vi "LV_webcam_image_analysis.vi"() -> ()   [LabVIEW 2014]
uses:
  <vilib>/userdefined/High Color/IMAQdx.ctl
  <vilib>/vision/driver/NI_Vision_Acquisition_Software.lvlib
  <vilib>/vision/NI_Vision_Development_Module.lvlib
panel:
  out "Boolean 2":bool
  out "Boolean":bool
  out "Color Spectrum":dbl[](array[numeric]) format="%.2f"
  out "Image":T1(plugin-control)
  in  "Stop Button":bool
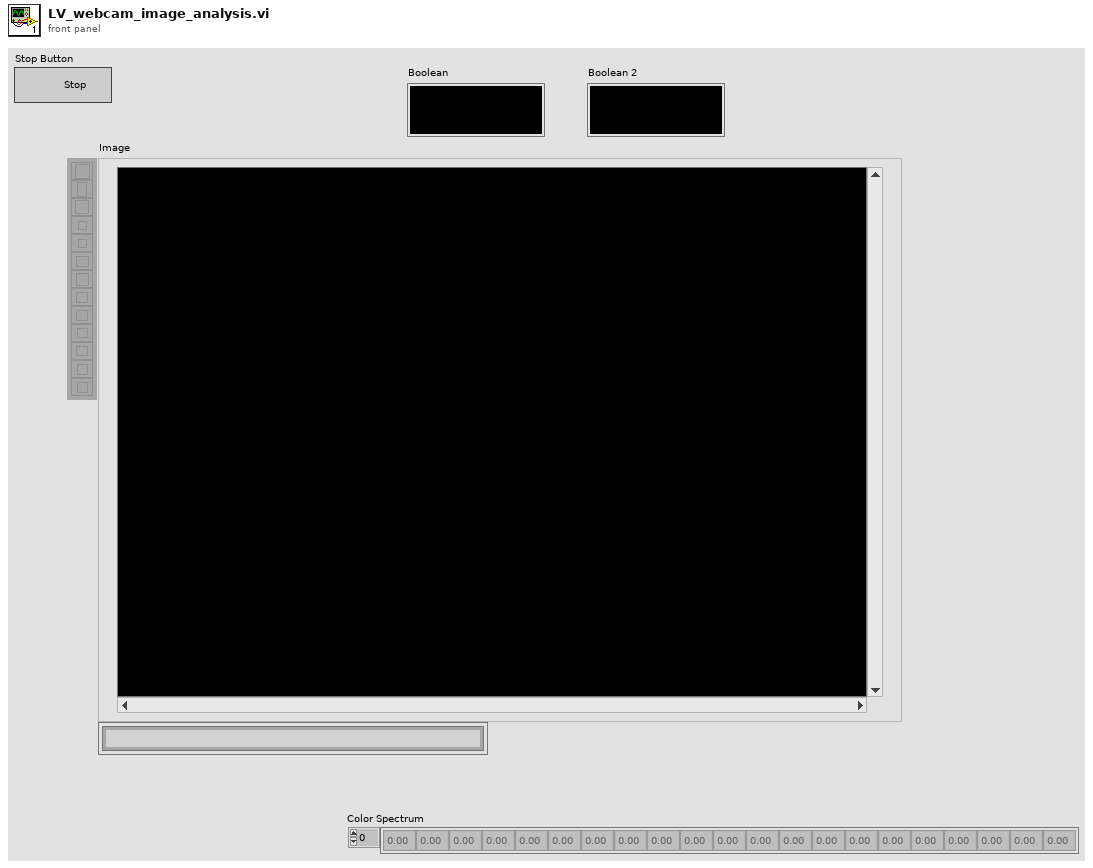
[diagram p1: front panel]
types:
  T1 = typedef "IMAQ Image.ctl" = refnum<image>
  T2 = typedef "IMAQdx.ctl" = refnum<k21>
  T3 = cluster{"Global Rectangle":i32[], "Contours":cluster{"Contour Type":u32, "ROI Type":u32, "Points":i32[]}[]}
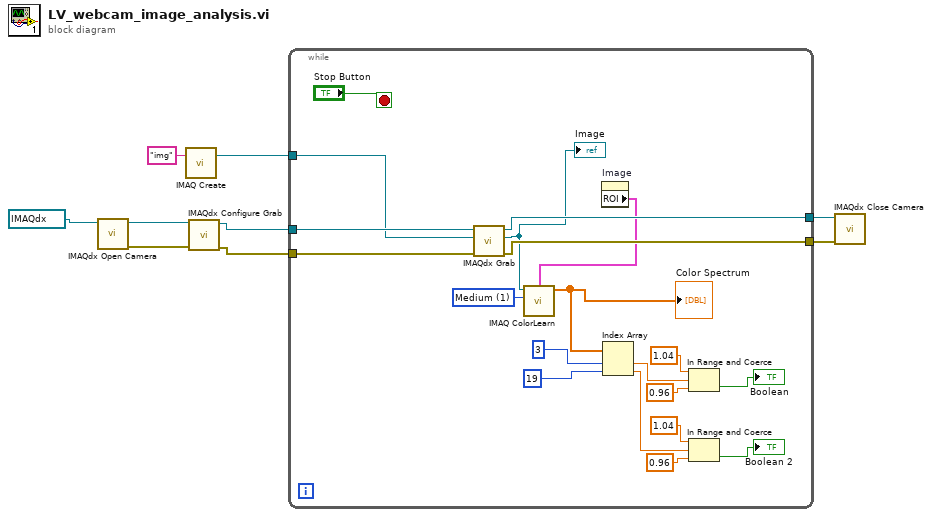
[diagram p0: block diagram]
diagram:
  n1 = call <vilib>:"IMAQdx Open Camera.vi"("Session In"=T2 "cam0") -> ("error out"=w9:errorcluster, "Session Out"=w6:T2)  [unwired: 9 in]
  n2 = call "IMAQ Create"("Image Name"="img") -> ("New Image"=w2:T1)  [unwired: 4 in, 1 out]
  n3 = call <vilib>:"IMAQdx Configure Grab.vi"("error in"=w9, "Session In"=w6) -> ("error out"=w8:errorcluster, "Session Out"=w5:T2)  [unwired: 8 in]
  n4 = while {
    tunnel: w8 -> [w28]
    tunnel: [w27] -> w7
    tunnel: w5 -> [w26]
    tunnel: [w25] -> w4
    tunnel: w2 -> [w24]
    stop <- "Stop Button" stop-if-true
    w22 = u32 1 items=["Low", "Medium", "High"] ("Color Sensitivity")
    n5 = call <vilib>:"IMAQdx Grab.vi"("error in"=w28, "Image In"=w24, "Session In"=w26) -> ("error out"=w27:errorcluster, "Image Out"=w23:T1, "Session Out"=w25:T2)  [unwired: 5 in, 1 out]
    "Image" <- w23
    n6 = property on="Image" class="ImageControl"() -> ("ROI"=w21:T3)  [unwired: 2 in, 2 out]
    n7 = call "IMAQ ColorLearn"("ROI Descriptor"=w21, "Image"=w23, "Color Sensitivity"=w22) -> ("Color Spectrum"=w20:dbl[])  [unwired: 5 in, 1 out]
    "Color Spectrum" <- w20
    n8 = Index Array(array=w20, index #1=3 ("index"), index #2=19 ("index")) -> (element #1=w18:dbl, element #2=w10:dbl)
    n9 = In Range and Coerce(upper limit=1.04, x=w18, lower limit=0.96) -> (In Range?=→"Boolean":bool)  [unwired: 1 out]
    n10 = In Range and Coerce(upper limit=1.04, x=w10, lower limit=0.96) -> (In Range?=→"Boolean 2":bool)  [unwired: 1 out]
  }
  n11 = call <vilib>:"IMAQdx Close Camera.vi"("error in"=w7, "Session In"=w4) -> ()  [unwired: 9 in, 1 out]
